vi "HFRR ADV v024 new software.vi"() -> ()   [LabVIEW 2025] (continued)
                n264 = local write "measured_stroke"(0.0 ("measured_stroke")) -> ()
                n265 = local write "Main Dashboard Buttons"(T1."Imaging" ("Main Dashboard Buttons")) -> ()
                n266 = property on="RUN" class="Bool (strict)"("Visible"=TRUE) -> ()  [unwired: 2 in, 2 out]
                n267 = local write "Due Write"("VC;0") -> ()
                n268 = local write "TEST FILE NAM,E SAVED"(FALSE ("TEST FILE NAM,E SAVED")) -> ()
                n269 = local write "Fuel Discription :"(w365) -> ()
                n270 = local write "Batch Ref Num :"(w365) -> ()
                n271 = local write "Remarks :"(w365) -> ()
                n272 = local write "FILE"(w365) -> ()
                n273 = property on="FRICVALZ 2" class="Bool (strict)"("DisabledEnum"=w364) -> ()  [unwired: 2 in, 2 out]
                n274 = property on="FRICVALZ 4" class="Bool (strict)"("DisabledEnum"=w364) -> ()  [unwired: 2 in, 2 out]
                n275 = property on="FRICVALZ 3" class="Bool (strict)"("DisabledEnum"=w364) -> ()  [unwired: 2 in, 2 out]
              }
            }
          }
          frame True {
            n276 = flat-sequence {
              frame #0 {
                n277 = local write "Due Write"("VC;1") -> ()
              }
              frame #1 {
                n278 = Wait (ms)(milliseconds to wait=u32 2000) -> ()  [unwired: 1 out]
              }
              frame #2 {
                n279 = local write "Due Write"("VC;1") -> ()
              }
              frame #3 {
                n280 = Wait (ms)(milliseconds to wait=u32 2000) -> ()  [unwired: 1 out]
              }
              frame #4 {
                w372 = T19."Disabled" ("Disabled")
                n281 = property on="RUN" class="Bool (strict)"("Visible"=FALSE) -> ()  [unwired: 2 in, 2 out]
                n282 = property on="FRICVALZ 2" class="Bool (strict)"("DisabledEnum"=w372) -> ()  [unwired: 2 in, 2 out]
                n283 = property on="FRICVALZ 4" class="Bool (strict)"("DisabledEnum"=w372) -> ()  [unwired: 2 in, 2 out]
                n284 = property on="FRICVALZ 3" class="Bool (strict)"("DisabledEnum"=w372) -> ()  [unwired: 2 in, 2 out]
                "START TEMP" <- TRUE
              }
            }
          }
        }
      }
      event "FILE", "USERNAME", "USER ID": Mouse Enter {
        n285 = event-data() -> ()  [unwired: 1 in, 4 out]
        n286 = dll-call lib="kernel32.dll" fn="Wow64DisableWow64FsRedirection"("OldValue"=0) -> (error out=w379:errorcluster, "OldValue"=w377:i32)  [unwired: 4 in, 1 out]
        n287 = call <vilib>:"System Exec.vi"("run minimized? (F)"=TRUE, "error in (no error)"=w379, "command line"="C:\\Program Files\\Common Files\\Microsoft Shared\\Ink\\TabTip.exe") -> ("error out"=w378:errorcluster)  [unwired: 5 in, 3 out]
        n288 = dll-call lib="kernel32.dll" fn="Wow64EnableWow64FsRedirection"(error in=w378, "OldValue"=w377) -> ()  [unwired: 4 in, 2 out]
      }
      event "EDIT": Value Change {
        n289 = event-data() -> ()  [unwired: 1 in, 6 out]
        n290 = local read "EDIT"() -> (w380:bool)
        n291 = case shown="False" w380 {
          frame False {
            n292 = control-ref of="This VI"() -> (w397:refnum<vi>)
            n293 = property class="VI"(reference=w397) -> (reference out=w388:refnum<vi>, error out=w392:errorcluster, "Panel"=w396:refnum<vi>)  [unwired: 1 in]
            n294 = property class="Pnl"(reference=w396, error in=w392) -> (reference out=w390:refnum<vi>, error out=w393:errorcluster, "Panes[]"=w395:refnum<vi>[])
            n295 = for {
              tunnel: w395 -> [w403] mode=indexing
              tunnel: T21."Always Off" ("Horizontal Scrollbar Visibility") -> [w402]
              tunnel: w393 -> [w399]
              tunnel: [w398] -> w391
              n296 = property class="Pane"(reference=w403, error in=w399, "HorizScrollbarVisibility"=w402) -> (reference out=w400:refnum<vi>, error out=w401:errorcluster)
              n297 = Close Reference(reference=w400, error in (no error)=w401) -> (error out=w398:errorcluster)
            }
            n298 = Close Reference(reference=w390, error in (no error)=w391) -> (error out=w389:errorcluster)
            n299 = Close Reference(reference=w388, error in (no error)=w389) -> (error out=w383:errorcluster)
            "error out 7" <- w383
            n300 = call <vilib>:"Clear Errors.vi"("error in (no error)"=w383) -> ("error out"=w382:errorcluster)  [unwired: 5 in, 1 out]
            n301 = local write "Service Password enable"(FALSE ("Service Password enable")) -> ()
            n302 = call <userlib>:"Fit VI window to Largest Dec.vi"("error in (no error)"=w382, "border spacing (2 px)"=1) -> ("error out"=w387:errorcluster, "dup VI Ref"=w385:refnum<vi>)  [unwired: 4 in]
            n303 = invoke on="Invoke Node" class="VI" method="FP.Run-Time Position.Maximized"(reference=w385, error in=w387) -> (error out=w386:errorcluster)  [unwired: 2 in, 3 out]
            n304 = call <vilib>:"Clear Errors.vi"("error in (no error)"=w386) -> ()  [unwired: 5 in, 2 out]
          }
          frame True {
          }
        }
      }
      event "Heater Button": Value Change {
        n305 = event-data() -> ()  [unwired: 1 in, 6 out]
        n306 = local read "Heater Button"() -> (w404:bool)
        n307 = case shown="True" w404 {
          frame True {
            n308 = stacked-sequence {
              frame #0 {
                n309 = Wait (ms)(milliseconds to wait=u32 1500) -> ()  [unwired: 1 out]
              }
              frame #1 {
                n310 = local read "Set Temp"() -> (w406:dbl)
                n311 = Number To Fractional String(number=w406, precision (6)=i16 2) -> (F-format string=w409:string)  [unwired: 2 in]
                n312 = Concatenate Strings("ST;" ("Command"), w409) -> (w408:string)
                n313 = local write "Due Write"(w408) -> ()
              }
              frame #2 {
                n314 = Wait (ms)(milliseconds to wait=u32 1500) -> ()  [unwired: 1 out]
              }
              frame #3 {
                n315 = local write "Due Write"("HE;1" ("Command")) -> ()
              }
              frame #4 {
                n316 = Wait (ms)(milliseconds to wait=u32 1500) -> ()  [unwired: 1 out]
              }
              frame #5 {
                n317 = stacked-sequence {
                  frame #0 {
                    n318 = Wait (ms)(milliseconds to wait=u32 1500) -> ()  [unwired: 1 out]
                  }
                  frame #1 {
                    n319 = local read "Set Temp"() -> (w415:dbl)
                    n320 = Number To Fractional String(number=w415, precision (6)=i16 2) -> (F-format string=w418:string)  [unwired: 2 in]
                    n321 = Concatenate Strings("ST;" ("Command"), w418) -> (w417:string)
                    n322 = local write "Due Write"(w417) -> ()
                  }
                  frame #2 {
                    n323 = Wait (ms)(milliseconds to wait=u32 1500) -> ()  [unwired: 1 out]
                  }
                  frame #3 {
                    n324 = local write "Due Write"("HE;1" ("Command")) -> ()
                  }
                  frame #4 {
                    n325 = Wait (ms)(milliseconds to wait=u32 1500) -> ()  [unwired: 1 out]
                  }
                }
              }
            }
          }
          frame False {
            n326 = stacked-sequence {
              frame #0 {
                n327 = Wait (ms)(milliseconds to wait=u32 1500) -> ()  [unwired: 1 out]
              }
              frame #1 {
                n328 = Concatenate Strings("ST;" ("Command"), "0" ("string")) -> (w425:string)
                n329 = local write "Due Write"(w425) -> ()
              }
              frame #2 {
                n330 = Wait (ms)(milliseconds to wait=u32 1500) -> ()  [unwired: 1 out]
              }
              frame #3 {
                n331 = local write "Due Write"("HE;0" ("Command")) -> ()
              }
              frame #4 {
                n332 = Wait (ms)(milliseconds to wait=u32 1500) -> ()  [unwired: 1 out]
              }
            }
          }
        }
      }
      event "Headen Service Button": Value Change {
        n333 = event-data() -> ()  [unwired: 1 in, 6 out]
        n334 = local read "Headen Service Button"() -> (w430:bool)
        n335 = case shown="True" w430 {
          frame False {
            n336 = property on="Password 3" class="Clust (strict)"("Visible"=FALSE) -> ()  [unwired: 2 in, 2 out]
            n337 = property on="Service Password Log" class="Str"("Visible"=FALSE) -> ()  [unwired: 2 in, 2 out]
          }
          frame True {
            n338 = property on="Password 3" class="Clust (strict)"("Visible"=TRUE) -> ()  [unwired: 2 in, 2 out]
            n339 = property on="Service Password Log" class="Str"("Visible"=TRUE) -> ()  [unwired: 2 in, 2 out]
          }
        }
      }
      event "Password 3.Service Password": Value Change {
        n340 = event-data() -> ()  [unwired: 1 in, 6 out]
        n341 = Unbundle By Name("Password 3") -> ("Service Password"=w437:string)
        n342 = call <vilib>:"Trim Whitespace.vi"("string"=w437) -> ("trimmed string"=w435:string)  [unwired: 1 in]
        n343 = Equal?(x=w435, y="Service@123") -> (x = y?=w436:bool)
        n344 = case shown="False" w436 {
          selector: w436 -> [w441 w443]
          frame False {
            n345 = local write "Service Password enable"(w441) -> ()
            n346 = property on="Service Password Log" class="Str"("Visible"=TRUE) -> ()  [unwired: 2 in, 2 out]
            n347 = property on="Tab Control 5" class="TabCtl (strict)"("Tabs Visible?"=TRUE ("Page Labels Display Visible?")) -> ()  [unwired: 2 in, 2 out]
          }
          frame True {
            n348 = property on="Service Password Log" class="Str"("Visible"=FALSE) -> ()  [unwired: 2 in, 2 out]
            "Service Password enable" <- w443
          }
        }
      }
      event "Sign In": Value Change {
        w445 = FALSE ("Visible")
        n349 = event-data() -> ()  [unwired: 1 in, 6 out]
        n350 = property on="About" class="Clust (strict)"("Visible"=w445) -> ()  [unwired: 2 in, 2 out]
        n351 = property on="Password 3" class="Clust (strict)"("Visible"=w445) -> ()  [unwired: 2 in, 2 out]
        n352 = property on="Service Password Log" class="Str"("Visible"=FALSE) -> ()  [unwired: 2 in, 2 out]
      }
      event "Info": Value Change {
        n353 = event-data() -> ()  [unwired: 1 in, 6 out]
        n354 = local read "Info"() -> (w447:bool)
        n355 = case shown="False" w447 {
          frame False {
            n356 = property on="About" class="Clust (strict)"("Visible"=FALSE) -> ()  [unwired: 2 in, 2 out]
          }
          frame True {
            n357 = property on="About" class="Clust (strict)"("Visible"=TRUE) -> ()  [unwired: 2 in, 2 out]
          }
        }
      }
      event "Calibration": Value Change {
        n358 = event-data() -> ()  [unwired: 1 in, 6 out]
        n359 = local read "Calibration"() -> (w451:bool)
        n360 = case shown="False" w451 {
          frame False {
            n361 = property on="Calibration 2" class="TabCtl (strict)"("Visible"=FALSE) -> ()  [unwired: 2 in, 2 out]
            n362 = local write "Cal Password"("" ("Cal Password")) -> ()
          }
          frame True {
            n363 = property on="Calibration 2" class="TabCtl (strict)"("Visible"=TRUE) -> ()  [unwired: 2 in, 2 out]
            n364 = local write "Cal Password"("" ("Cal Password")) -> ()
          }
        }
        n365 = property on="Wrong Password" class="Str"("Visible"=FALSE) -> ()  [unwired: 2 in, 2 out]
      }
      event "Cal Password": Value Change {
        n366 = event-data() -> ()  [unwired: 1 in, 6 out]
        n367 = local read "Cal Password"() -> (w459:string)
        n368 = call <vilib>:"Trim Whitespace.vi"("string"=w459) -> ("trimmed string"=w458:string)  [unwired: 1 in]
        n369 = Equal?(x=w458, y="Cal@321") -> (x = y?=w456:bool)
        n370 = case shown="True" w456 {
          frame False {
            n371 = property on="Wrong Password" class="Str"("Visible"=TRUE) -> ()  [unwired: 2 in, 2 out]
          }
          frame True {
            n372 = property on="Wrong Password" class="Str"("Visible"=FALSE) -> ()  [unwired: 2 in, 2 out]
            n373 = local write "Main Tab"(T2."About" ("Main Tab")) -> ()
            n374 = local write "Cal Password"("" ("Cal Password")) -> ()
            n375 = local write "Main Dashboard Buttons"(T1."About" ("Main Dashboard Buttons")) -> ()
            n376 = local write "Tab Control 5"(T12."Temperature Calibration" ("Tab Control 5")) -> ()
            n377 = property on="Calibration 2" class="TabCtl (strict)"("Visible"=FALSE) -> ()  [unwired: 2 in, 2 out]
            n378 = property on="Tab Control 5" class="TabCtl (strict)"("Tabs Visible?"=FALSE ("Page Labels Display Visible?")) -> ()  [unwired: 2 in, 2 out]
            n379 = local write "Calibration"(FALSE ("Calibration")) -> ()
          }
        }
      }
      event "Calibration Selection": Value Change {
        n380 = event-data() -> ()  [unwired: 1 in, 6 out]
        n381 = local read "Calibration Selection"() -> (w470:T8)
        n382 = case shown="\"Stroke Calibration\"" w470 {
          tunnel: [T7."Stroke" ("Main Calibration Tab") T7."Friction" ("Main Calibration Tab") T7."Main" ("Main Calibration Tab") T7."Temperature" ("Main Calibration Tab")] -> w469
          frame "Stroke Calibration" {
          }
          frame "Friction Force Calibration" {
          }
          frame Default {
          }
          frame "Temperature Calibration" {
          }
        }
        n383 = local write "Main Calibration Tab"(w469) -> ()
      }
      event "Back Stroke": Value Change {
        n384 = event-data() -> ()  [unwired: 1 in, 6 out]
        n385 = local write "Main Stroke Tab"(T9."Step 1" ("Main Stroke Tab")) -> ()
        n386 = local write "Main Calibration Tab"(T7."Main" ("Main Calibration Tab")) -> ()
        n387 = local write "Back Stroke"(FALSE ("Back Stroke")) -> ()
      }
      event "Step 2 Back": Value Change {
        n388 = event-data() -> ()  [unwired: 1 in, 6 out]
        n389 = local write "Main Stroke Tab"(T9."Step 1" ("Main Stroke Tab")) -> ()
        n390 = local write "Step 2 Back"(FALSE ("Back Stroke")) -> ()
      }
      event "Step 3 Back": Value Change {
        n391 = event-data() -> ()  [unwired: 1 in, 6 out]
        n392 = local write "Main Stroke Tab"(T9."Step 2" ("Main Stroke Tab")) -> ()
        n393 = local write "Step 3 Back"(FALSE ("Back Stroke")) -> ()
      }
      event "Step 4 Back": Value Change {
        n394 = event-data() -> ()  [unwired: 1 in, 6 out]
        n395 = local write "Main Stroke Tab"(T9."Step 3" ("Main Stroke Tab")) -> ()
        n396 = local write "Step 4 Back"(FALSE ("Back Stroke")) -> ()
      }
      event "Step 5 Back": Value Change {
        n397 = event-data() -> ()  [unwired: 1 in, 6 out]
        n398 = local write "Main Stroke Tab"(T9."Step 4" ("Main Stroke Tab")) -> ()
        n399 = local write "Step 5 Back"(FALSE ("Back Stroke")) -> ()
      }
      event "Step 6 Back": Value Change {
        n400 = event-data() -> ()  [unwired: 1 in, 6 out]
        n401 = local write "Main Stroke Tab"(T9."Step 5" ("Main Stroke Tab")) -> ()
        n402 = local write "Step 6 Back"(FALSE ("Back Stroke")) -> ()
      }
      event "Back Stroke step 7": Value Change {
        n403 = event-data() -> ()  [unwired: 1 in, 6 out]
        n404 = local write "Main Stroke Tab"(T9."Step 6" ("Main Stroke Tab")) -> ()
        n405 = local write "Back Stroke step 7"(FALSE ("Back Stroke")) -> ()
      }
      event "Back Stroke step 8": Value Change {
        n406 = event-data() -> ()  [unwired: 1 in, 6 out]
        n407 = local write "Main Stroke Tab"(T9."Step 7" ("Main Stroke Tab")) -> ()
        n408 = local write "Back Stroke step 8"(FALSE ("Back Stroke")) -> ()
      }
      event "Back Stroke 8": Value Change {
        n409 = event-data() -> ()  [unwired: 1 in, 6 out]
        n410 = local write "MOVE CARRIAGE TO"(0.2 ("MOVE CARRIAGE TO")) -> ()
        n411 = local write "Main Stroke Tab"(T9."Step 1" ("Main Stroke Tab")) -> ()
        n412 = local write "Back Stroke 8"(FALSE ("Back Stroke 8")) -> ()
      }
      event "Continue Stroke": Value Change {
        n413 = event-data() -> ()  [unwired: 1 in, 6 out]
        n414 = local write "Main Stroke Tab"(T9."Step 2" ("Main Stroke Tab")) -> ()
        n415 = local write "Continue Stroke"(FALSE ("Continue Stroke")) -> ()
      }
      event "Continue Stroke step 2": Value Change {
        n416 = event-data() -> ()  [unwired: 1 in, 6 out]
        n417 = local write "Main Stroke Tab"(T9."Step 3" ("Main Stroke Tab")) -> ()
        n418 = local write "Continue Stroke step 2"(FALSE ("Continue Stroke")) -> ()
      }
      event "Continue Stroke step 3": Value Change {
        n419 = event-data() -> ()  [unwired: 1 in, 6 out]
        n420 = local write "Main Stroke Tab"(T9."Step 4" ("Main Stroke Tab")) -> ()
        n421 = local write "Continue Stroke step 3"(FALSE ("Continue Stroke")) -> ()
      }
      event "Continue Stroke step 4": Value Change {
        n422 = event-data() -> ()  [unwired: 1 in, 6 out]
        n423 = local write "Main Stroke Tab"(T9."Step 5" ("Main Stroke Tab")) -> ()
        n424 = local write "Continue Stroke step 4"(FALSE ("Continue Stroke")) -> ()
      }
      event "Continue Stroke step 5": Value Change {
        n425 = event-data() -> ()  [unwired: 1 in, 6 out]
        n426 = local write "Main Stroke Tab"(T9."Step 6" ("Main Stroke Tab")) -> ()
        n427 = local write "Continue Stroke step 5"(FALSE ("Continue Stroke")) -> ()
      }
      event "Continue Stroke step 6": Value Change {
        n428 = event-data() -> ()  [unwired: 1 in, 6 out]
        n429 = local write "Main Stroke Tab"(T9."Step 7" ("Main Stroke Tab")) -> ()
        n430 = local write "Continue Stroke step 6"(FALSE ("Continue Stroke")) -> ()
      }
      event "Continue Stroke step 7": Value Change {
        w509 = FALSE ("0.2mm")
        n431 = event-data() -> ()  [unwired: 1 in, 6 out]
        n432 = local write "0.4 mm"(w509) -> ()
        n433 = local write "0.6 mm"(w509) -> ()
        n434 = local write "1.0 mm"(w509) -> ()
        n435 = local write "1.2 mm"(w509) -> ()
        n436 = local write "0.2 2"(w509) -> ()
        n437 = local write "0.4 2"(w509) -> ()
        n438 = local write "0.6 2"(w509) -> ()
        n439 = local write "0.8 2"(w509) -> ()
        n440 = local write "1.0 2"(w509) -> ()
        n441 = local write "1.2"(w509) -> ()
        n442 = local write "0.2mm"(w509) -> ()
        n443 = local write "0.8mm"(w509) -> ()
        n444 = local write "Main Stroke Tab"(T9."Step 8" ("Main Stroke Tab")) -> ()
        n445 = local write "Continue Stroke step 7"(FALSE ("Continue Stroke")) -> ()
        n446 = local write "Stroke Test Complete"(T10."Test Progress" ("Stroke Test Complete")) -> ()
        "Position Measurment Temp" <- 0.0 ("Position Measurment Temp")
        "Calibration Tare" <- TRUE ("Calibration Tare")
        "MOVE CARRIAGE TO" <- 0.2 ("MOVE CARRIAGE TO")
      }
      event "Continue Stroke step 8": Value Change {
        n447 = event-data() -> ()  [unwired: 1 in, 6 out]
        n448 = local read "LVDT STROKE  Calibration"() -> (w514:dbl)
        n449 = local read "Position Measurment Temp"() -> (w515:dbl)
        n450 = case shown="7" w515 {
          selector: w515 -> [w520 w525 w530 w535 w540 w544 w547 w548]
          tunnel: w514 -> [w516 w521 w526 w531 w536 w541 _ _]
          frame 0, Default {
            w518 = TRUE ("0.2mm")
            n451 = Increment(x=w520) -> (x+1=w519:i32)
            n452 = local write "Position Measurment Temp"(w519) -> ()
            n453 = local write "0.2mm"(w518) -> ()
            n454 = local write "0.2 2"(w518) -> ()
            n455 = local write "MOVE CARRIAGE TO"(0.4 ("MOVE CARRIAGE TO")) -> ()
            "Calibration 0.2" <- w516
          }
          frame 1 {
            w523 = TRUE ("0.4 mm")
            n456 = Increment(x=w525) -> (x+1=w524:i32)
            n457 = local write "Calibration 0.4"(w521) -> ()
            n458 = local write "Position Measurment Temp"(w524) -> ()
            n459 = local write "0.4 mm"(w523) -> ()
            n460 = local write "MOVE CARRIAGE TO"(0.6 ("MOVE CARRIAGE TO")) -> ()
            n461 = local write "0.4 2"(w523) -> ()
          }
          frame 2 {
            w528 = TRUE ("0.6 mm")
            n462 = Increment(x=w530) -> (x+1=w529:i32)
            n463 = local write "Calibration 0.6"(w526) -> ()
            n464 = local write "Position Measurment Temp"(w529) -> ()
            n465 = local write "0.6 2"(w528) -> ()
            n466 = local write "0.6 mm"(w528) -> ()
            n467 = local write "MOVE CARRIAGE TO"(0.8 ("MOVE CARRIAGE TO")) -> ()
          }
          frame 3 {
            w532 = TRUE ("0.6 mm")
            n468 = Increment(x=w535) -> (x+1=w534:i32)
            n469 = local write "Position Measurment Temp"(w534) -> ()
            n470 = local write "MOVE CARRIAGE TO"(1.0 ("MOVE CARRIAGE TO")) -> ()
            n471 = local write "0.8mm"(w532) -> ()
            n472 = local write "0.8 2"(w532) -> ()
            "Calibration 0.8" <- w531
          }
          frame 4 {
            w537 = TRUE ("0.6 mm")
            n473 = Increment(x=w540) -> (x+1=w539:i32)
            n474 = local write "Position Measurment Temp"(w539) -> ()
            n475 = local write "MOVE CARRIAGE TO"(1.2 ("MOVE CARRIAGE TO")) -> ()
            n476 = local write "1.0 mm"(w537) -> ()
            n477 = local write "1.0 2"(w537) -> ()
            "Calibration 1.0" <- w536
          }
          frame 5 {
            w542 = TRUE ("0.6 mm")
            n478 = Increment(x=w544) -> (x+1=w543:i32)
            n479 = local write "Position Measurment Temp"(w543) -> ()
            n480 = local write "1.2 mm"(w542) -> ()
            n481 = local write "1.2"(w542) -> ()
            "Calibration 1.2" <- w541
          }
          frame 6 {
            n482 = Increment(x=w547) -> (x+1=w546:i32)
            n483 = local write "Position Measurment Temp"(w546) -> ()
            n484 = local write "Stroke Test Complete"(T10."Stroke Points Completed" ("Stroke Test Complete")) -> ()
          }
          frame 7 {
            n485 = stacked-sequence {
              tunnel: w548 -> [w549 _ _]
              frame #0 {
                n486 = Increment(x=w549) -> (x+1=w550:i32)
                n487 = local write "Main Stroke Tab"(T9."Step 9" ("Main Stroke Tab")) -> ()
                n488 = local write "Position Measurment Temp"(w550) -> ()
                n489 = Insert Into Array(array=dbl[] [], new element #1=0.2 ("new element/subarray"), new element #2=0.4 ("new element/subarray"), new element #3=0.6 ("new element/subarray"), new element #4=0.8 ("new element/subarray"), new element #5=1.0 ("new element/subarray"), new element #6=1.2 ("new element/subarray")) -> (→"1D stroke":dbl[])  [unwired: 1 in]
                n490 = local read "Calibration 0.2"() -> (w557:dbl)
                n491 = local read "Calibration 0.4"() -> (w556:dbl)
                n492 = local read "Calibration 0.6"() -> (w555:dbl)
                n493 = local read "Calibration 0.8"() -> (w554:dbl)
                n494 = local read "Calibration 1.0"() -> (w553:dbl)
                n495 = local read "Calibration 1.2"() -> (w552:dbl)
                n496 = Insert Into Array(array=dbl[] [], new element #1=w557, new element #2=w556, new element #3=w555, new element #4=w554, new element #5=w553, new element #6=w552) -> (→"Calibrated Voltage Value":dbl[])  [unwired: 1 in]
              }
              frame #1 {
                n497 = local read "calibration values"() -> (w580:dbl[])
                n498 = local read "Calibrated Voltage Value"() -> (w582:dbl[])
                n499 = Index Array(array=w580, index #1=1 ("index"), index #2=3 ("index"), index #3=5 ("index"), index #4=7 ("index"), index #5=9 ("index"), index #6=11 ("index")) -> (element #1=w573:dbl, element #2=w572:dbl, element #3=w571:dbl, element #4=w570:dbl, element #5=w569:dbl, element #6=w568:dbl)
                n500 = local read "1D stroke"() -> (w583:dbl[])
                n501 = for {
                  tunnel: [w592] -> w581 mode=indexing
                  tunnel: w583 -> [w591] mode=indexing
                  tunnel: w582 -> [w590] mode=indexing
                  tunnel: w573 -> [w589]
                  tunnel: w572 -> [w588]
                  tunnel: w571 -> [w587]
                  tunnel: w570 -> [w586]
                  tunnel: w569 -> [w585]
                  tunnel: w568 -> [w584]
                  n502 = formula code="if (stroke == 0.2)\n{\n    if ((voltage >= REF_02 * 0.985) && (voltage <= REF_02 * 1.015))\n        status = 1;\n    else\n        status = 0;\n}\nelse if (stroke == 0.4)\n{\n    if ((voltage >= REF_04 * 0.985) && (voltage <= REF_04 * 1.015))\n        status = 1;\n    else\n        status = 0;\n}\nelse if (stroke == 0.6)\n{\n    if ((voltage >= REF_06 * 0.985) && (voltage <= REF_06 * 1.015))\n        status = 1;\n    else\n        status = 0;\n}\nelse if (stroke == 0.8)\n{\n    if ((voltage >= REF_08 * 0.985) && (voltage <= REF_08 * 1.015))\n        status = 1;\n    else\n        status = 0;\n}\nelse if (stroke == 1.0)\n{\n    if ((voltage >= REF_10 * 0.985) && (voltage <= REF_10 * 1.015))\n        status = 1;\n    else\n        status = 0;\n}\nelse if (stroke == 1.2)\n{\n    if ((voltage >= REF_12 * 0.985) && (voltage <= REF_12 * 1.015))\n        status = 1;\n    else\n        status = 0;\n}\nelse\n{\n    status = 0;\n}"("stroke"=w591, "voltage"=w590, "REF_02"=w589, "REF_04"=w588, "REF_06"=w587, "REF_08"=w586, "REF_10"=w585, "REF_12"=w584) -> ("status"=w592:dbl)
                }
                "Status" <- w581
              }
              frame #2 {
                w599 = 1.0
                n503 = local read "Status"() -> (w606:dbl[])
                n504 = Index Array(array=w606) -> (element #1=w605:dbl, element #2=w604:dbl, element #3=w603:dbl, element #4=w602:dbl, element #5=w601:dbl, element #6=w600:dbl)  [unwired: 6 in]
                n505 = Equal?(x=w604, y=w599) -> (x = y?=w597:bool)
                n506 = Equal?(x=w603, y=w599) -> (x = y?=w596:bool)
                n507 = Equal?(x=w602, y=w599) -> (x = y?=w595:bool)
                n508 = Equal?(x=w601, y=w599) -> (x = y?=w594:bool)
                n509 = Equal?(x=w600, y=w599) -> (x = y?=w593:bool)
                n510 = Equal?(x=w605, y=w599) -> (x = y?=w598:bool)
                n511 = case shown="True" w598 {
                  selector: w598 -> [w617 w618]
                  frame True {
                    n512 = local write "Point 1 - 0.2 mm"(w617) -> ()
                    n513 = property on="Point 1 - 0.2 mm" class="Bool"("Caption.Visible"=w617) -> ()  [unwired: 2 in, 2 out]
                  }
                  frame False {
                    n514 = local write "Point 1 - 0.2 mm"(w618) -> ()
                    n515 = property on="Point 1 - 0.2 mm" class="Bool"("Caption.Visible"=w618) -> ()  [unwired: 2 in, 2 out]
                  }
                }
                n516 = case shown="True" w597 {
                  selector: w597 -> [w615 w616]
                  frame True {
                    n517 = local write "Point 2 - 0.4 mm"(w615) -> ()
                    n518 = property on="Point 2 - 0.4 mm" class="Bool"("Caption.Visible"=w615) -> ()  [unwired: 2 in, 2 out]
                  }
                  frame False {
                    n519 = local write "Point 2 - 0.4 mm"(w616) -> ()
                    n520 = property on="Point 2 - 0.4 mm" class="Bool"("Caption.Visible"=w616) -> ()  [unwired: 2 in, 2 out]
                  }
                }
                n521 = case shown="True" w594 {
                  selector: w594 -> [w609 w610]
                  frame True {
                    n522 = local write "Point 5 - 1.0 mm"(w609) -> ()
                    n523 = property on="Point 5 - 1.0 mm" class="Bool"("Caption.Visible"=w609) -> ()  [unwired: 2 in, 2 out]
                  }
                  frame False {
                    n524 = local write "Point 5 - 1.0 mm"(w610) -> ()
                    n525 = property on="Point 5 - 1.0 mm" class="Bool"("Caption.Visible"=w610) -> ()  [unwired: 2 in, 2 out]
                  }
                }
                n526 = case shown="True" w596 {
                  selector: w596 -> [w613 w614]
                  frame True {
                    n527 = local write "Point 3 - 0.6 mm"(w613) -> ()
                    n528 = property on="Point 3 - 0.6 mm" class="Bool"("Caption.Visible"=w613) -> ()  [unwired: 2 in, 2 out]
                  }
                  frame False {
                    n529 = local write "Point 3 - 0.6 mm"(w614) -> ()
                    n530 = property on="Point 3 - 0.6 mm" class="Bool"("Caption.Visible"=w614) -> ()  [unwired: 2 in, 2 out]
                  }
                }
                n531 = case shown="True" w595 {
                  selector: w595 -> [w611 w612]
                  frame True {
                    n532 = local write "Point 4 - 0.8 mm"(w611) -> ()
                    n533 = property on="Point 4 - 0.8 mm" class="Bool"("Caption.Visible"=w611) -> ()  [unwired: 2 in, 2 out]
                  }
                  frame False {
                    n534 = local write "Point 4 - 0.8 mm"(w612) -> ()
                    n535 = property on="Point 4 - 0.8 mm" class="Bool"("Caption.Visible"=w612) -> ()  [unwired: 2 in, 2 out]
                  }
                }
                n536 = case shown="True" w593 {
                  selector: w593 -> [w607 w608]
                  frame True {
                    n537 = local write "Point 6 - 1.2 mm"(w607) -> ()
                    n538 = property on="Point 6 - 1.2 mm" class="Bool"("Caption.Visible"=w607) -> ()  [unwired: 2 in, 2 out]
                  }
                  frame False {
                    n539 = local write "Point 6 - 1.2 mm"(w608) -> ()
                    n540 = property on="Point 6 - 1.2 mm" class="Bool"("Caption.Visible"=w608) -> ()  [unwired: 2 in, 2 out]
                  }
                }
              }
            }
          }
        }
      }
      event "TEMPERATURE STEP Back 1", "TEMPERATURE STEP Back air Temp": Value Change {
        n541 = event-data() -> ()  [unwired: 1 in, 6 out]
        n542 = stacked-sequence {
          frame #0 {
            n543 = local write "Main Calibration Tab"(T7."Main" ("Main Calibration Tab")) -> ()
          }
          frame #1 {
            n544 = Wait (ms)(milliseconds to wait=u32 1000) -> ()  [unwired: 1 out]
          }
          frame #2 {
            n545 = local write "Due Write"("CAL;END" ("Command")) -> ()
          }
          frame #3 {
            n546 = Wait (ms)(milliseconds to wait=u32 2000) -> ()  [unwired: 1 out]
          }
          frame #4 {
            n547 = local write "Due Write"("CAL;END" ("Command")) -> ()
          }
        }
      }
      event "Temperature Continue Step 1": Value Change {
        n548 = event-data() -> ()  [unwired: 1 in, 6 out]
        n549 = stacked-sequence {
          frame #0 {
            n550 = Wait (ms)(milliseconds to wait=u32 1500) -> ()  [unwired: 1 out]
          }
          frame #1 {
            n551 = local write "Due Write"("CAL;START" ("Command")) -> ()
          }
          frame #2 {
            n552 = Wait (ms)(milliseconds to wait=u32 1500) -> ()  [unwired: 1 out]
          }
          frame #3 {
            n553 = local write "Due Write"("CAL;START" ("Command")) -> ()
          }
          frame #4 {
            n554 = Wait (ms)(milliseconds to wait=u32 2000) -> ()  [unwired: 1 out]
          }
          frame #5 {
          }
          frame #6 {
            n555 = Wait (ms)(milliseconds to wait=u32 2000) -> ()  [unwired: 1 out]
          }
          frame #7 {
            # "CAL;A1;<true_T>"
            n556 = local write "Due Write"("CAL;A1;0" ("Command")) -> ()
          }
          frame #8 {
            n557 = local write "Tab Control 4"(T11."Step 2" ("Tab Control 4")) -> ()
          }
        }
      }
      event "Temperature Continue Step air Step 1": Value Change {
        n558 = event-data() -> ()  [unwired: 1 in, 6 out]
        n559 = stacked-sequence {
          frame #0 {
            n560 = Wait (ms)(milliseconds to wait=u32 1500) -> ()  [unwired: 1 out]
          }
          frame #1 {
            n561 = local write "Due Write"("CAL;START" ("Command")) -> ()
          }
          frame #2 {
            n562 = local write "Tab Control 4"(T11."Air Step 2" ("Tab Control 4")) -> ()
            n563 = Wait (ms)(milliseconds to wait=u32 1500) -> ()  [unwired: 1 out]
          }
          frame #3 {
            n564 = local write "Due Write"("CAL;START" ("Command")) -> ()
          }
          frame #4 {
            n565 = Wait (ms)(milliseconds to wait=u32 2000) -> ()  [unwired: 1 out]
          }
          frame #5 {
            # "CAL;A1;<true_T>"
            n566 = local write "Due Write"("CAL;A2;0" ("Command")) -> ()
          }
          frame #6 {
            n567 = Wait (ms)(milliseconds to wait=u32 2000) -> ()  [unwired: 1 out]
          }
          frame #7 {
            # "CAL;A1;<true_T>"
            n568 = local write "Due Write"("CAL;A1;0" ("Command")) -> ()
          }
        }
      }
      event "Temperature Selection": Value Change {
        n569 = event-data() -> ()  [unwired: 1 in, 6 out]
        n570 = local read "Temperature Selection"() -> (w641:enum32{"Air Temperature", "Sample Temperature"})
        n571 = case shown="\"Sample Temperature\"" w641 {
          frame "Air Temperature", Default {
            n572 = local write "Tab Control 4"(T11."Air Step 1" ("Tab Control 4")) -> ()
          }
          frame "Sample Temperature" {
            n573 = local write "Tab Control 4"(T11."Step 1" ("Tab Control 4")) -> ()
          }
        }
      }
      event "Temperature Continue Step 2": Value Change {
        n574 = event-data() -> ()  [unwired: 1 in, 6 out]
        n575 = stacked-sequence {
          frame #0 {
            n576 = stacked-sequence {
              frame #0 {
                n577 = Wait (ms)(milliseconds to wait=u32 1500) -> ()  [unwired: 1 out]
              }
              frame #1 {
                # "CAL;A1;<true_T>"
                n578 = local write "Due Write"("CAL;A1;0" ("Command")) -> ()
              }
              frame #2 {
                n579 = Wait (ms)(milliseconds to wait=u32 1500) -> ()  [unwired: 1 out]
              }
              frame #3 {
                # "CAL;A1;<true_T>"
                n580 = local write "Due Write"("CAL;A1;0" ("Command")) -> ()
              }
              frame #4 {
              }
            }
          }
          frame #1 {
            n581 = local write "Tab Control 4"(T11."Step 3" ("Tab Control 4")) -> ()
          }
        }
      }
      event "Temperature Continue Step 3": Value Change {
        n582 = event-data() -> ()  [unwired: 1 in, 6 out]
        n583 = stacked-sequence {
          frame #0 {
            n584 = stacked-sequence {
              frame #0 {
                n585 = Wait (ms)(milliseconds to wait=u32 1500) -> ()  [unwired: 1 out]
              }
              frame #1 {
              }
              frame #2 {
              }
              frame #3 {
                # "CAL;A1;<true_T>"
                n586 = local write "Due Write"("CAL;A1;60" ("Command")) -> ()
              }
              frame #4 {
                n587 = Wait (ms)(milliseconds to wait=u32 2000) -> ()  [unwired: 1 out]
              }
              frame #5 {
                # "CAL;A1;<true_T>"
                n588 = local write "Due Write"("CAL;A1;60" ("Command")) -> ()
              }
            }
          }
          frame #1 {
            n589 = Wait (ms)(milliseconds to wait=u32 1000) -> ()  [unwired: 1 out]
          }
          frame #2 {
            n590 = local write "Due Write"("CAL;SAVE" ("Command")) -> ()
          }
          frame #3 {
            n591 = Wait (ms)(milliseconds to wait=u32 1000) -> ()  [unwired: 1 out]
          }
          frame #4 {
            n592 = local write "Due Write"("CAL;SAVE" ("Command")) -> ()
          }
          frame #5 {
            n593 = Wait (ms)(milliseconds to wait=u32 1000) -> ()  [unwired: 1 out]
          }
          frame #6 {
            # "CAL;END"
            n594 = local write "Due Write"("CAL;END" ("Command")) -> ()
          }
          frame #7 {
            n595 = Wait (ms)(milliseconds to wait=u32 1000) -> ()  [unwired: 1 out]
          }
          frame #8 {
            # "CAL;END"
            n596 = local write "Due Write"("CAL;END" ("Command")) -> ()
          }
          frame #9 {
            n597 = local write "Main Calibration Tab"(T7."Temperature" ("Main Calibration Tab")) -> ()
            n598 = local write "Tab Control 4"(T11."Main" ("Tab Control 4")) -> ()
          }
        }
      }
      event "Back Stroke step main temperature": Value Change {
        n599 = event-data() -> ()  [unwired: 1 in, 6 out]
        n600 = stacked-sequence {
          frame #0 {
            n601 = Wait (ms)(milliseconds to wait=u32 1000) -> ()  [unwired: 1 out]
          }
          frame #1 {
            # "CAL;END"
            n602 = local write "Due Write"("CAL;END" ("Command")) -> ()
          }
          frame #2 {
            n603 = Wait (ms)(milliseconds to wait=u32 1000) -> ()  [unwired: 1 out]
          }
          frame #3 {
            # "CAL;END"
            n604 = local write "Due Write"("CAL;END" ("Command")) -> ()
          }
          frame #4 {
            n605 = local write "Main Calibration Tab"(T7."Temperature" ("Main Calibration Tab")) -> ()
            n606 = local write "Tab Control 4"(T11."Main" ("Tab Control 4")) -> ()
          }
        }
      }
      event "Quit": Value Change {
        n607 = event-data() -> ()  [unwired: 1 in, 6 out]
      }
    }
    n608 = Wait (ms)(milliseconds to wait=u32 100) -> ()  [unwired: 1 out]
  }
  n609 = while {
    stop <- w674 stop-if-true
    n610 = local read "Ambient Temperature"() -> (w672:dbl)
    n611 = local read "Sample Temperature"() -> (w671:dbl)
    n612 = Wait (ms)(milliseconds to wait=u32 200) -> ()  [unwired: 1 out]
    n613 = local write "Temperature — Live (Set A: 0 °C)"(w672) -> ()
    n614 = local write "Temperature — Live (Set A: 60 °C)"(w672) -> ()
    n615 = local write "Sensor value"(w672) -> ()
    n616 = local write "Sensor value"(w672) -> ()
    n617 = local write "Sensor value"(w671) -> ()
    n618 = local write "Sensor value"(w671) -> ()
    n619 = local write "Temperature — Live (Set A: 60 °C)"(w671) -> ()
    n620 = local write "Temperature — Live (Set A: 60 °C)"(w671) -> ()
    n621 = case shown="True" "Save Button" {
      selector: "Save Button" -> [_ w676]
      frame False {
      }
      frame True {
        n622 = Not(x=w676) -> (.not. x?=w675:bool)
        n623 = local read "milliseconds to wait"() -> (w708:u32)
        n624 = local read "max_step_change"() -> (w713:dbl)
        n625 = local read "max_amplitude"() -> (w714:dbl)
        n626 = local read "min_amplitude"() -> (w715:dbl)
        n627 = local read "PIEZO_CAL_FACTOR"() -> (w719:dbl)
        n628 = local write "Save Button"(w675) -> ()
        n629 = local read "startup_cmd"() -> (w716:dbl)
        n630 = local read "NORMAL_FORCE"() -> (w720:dbl)
        n631 = local read "ADC_Resolution"() -> (w718:dbl)
        n632 = local read "calibration values"() -> (w723:dbl[])
        n633 = local read "kp"() -> (w710:dbl)
        n634 = local read "kd"() -> (w712:dbl)
        n635 = local read "dt"() -> (w709:dbl)
        n636 = local read "ki"() -> (w711:dbl)
        n637 = local read "STROKE FILTER"() -> (w721:i32)
        n638 = local read "Add up Stroke"() -> (w722:dbl)
        n639 = local read "VREF"() -> (w717:dbl)
        n640 = Insert Into Array(array=dbl[] [], new element #1=w708, new element #2=w709, new element #3=w710, new element #4=w711, new element #5=w712, new element #6=w713, new element #7=w714, new element #8=w715, new element #9=w716) -> (w724:dbl[])  [unwired: 1 in]
        n641 = Insert Into Array(array=dbl[] [], new element #1=w717, new element #2=w718, new element #3=w719, new element #4=w720) -> (w725:dbl[])  [unwired: 1 in]
        n642 = Array To Spreadsheet String(delimiter (Tab)=";", array=w723, 3:"" ("format string")) -> (spreadsheet string=w727:string)
        n643 = Insert Into Array(array=dbl[] [], new element #1=w721, new element #2=w722) -> (w726:dbl[])  [unwired: 1 in]
        n644 = call "Write Config.vi"("Stroke Calibration"=w727, "STROKE PARAMETERS"=w726, "ADC PARAMETERS"=w725, "PID  PARAMETERS"=w724) -> ("error out"=w706:errorcluster)  [unwired: 7 in]
        n645 = call "Stall Data Flow.vim"("value in"=w706, "milliseconds to wait"=u32 2000) -> ("value out"=w707:errorcluster)  [unwired: 1 out]
        n646 = call "Read Config.vi"("error in (no error)"=w707) -> ("STROKE PARAMETERS"=w704:dbl[], "ADC PARAMETERS"=w703:dbl[], "PID  PARAMETERS"=w702:dbl[], "Stroke Calibration"=w705:string)  [unwired: 6 in, 1 out]
        n647 = Index Array(array=w702) -> (element #1=w700:dbl, element #2=w699:dbl, element #3=w698:dbl, element #4=w697:dbl, element #5=w696:dbl, element #6=w695:dbl, element #7=w694:dbl, element #8=w693:dbl, element #9=w692:dbl)  [unwired: 9 in]
        n648 = Index Array(array=w703) -> (element #1=w691:dbl, element #2=w690:dbl, element #3=w689:dbl, element #4=w688:dbl)  [unwired: 4 in]
        n649 = Index Array(array=w704) -> (element #1=w687:dbl, element #2=w686:dbl)  [unwired: 2 in]
        n650 = Spreadsheet String To Array(delimiter (Tab)=";", format string="", spreadsheet string=w705, array type (2D Dbl)=dbl[] []) -> (array=w701:dbl[])
        n651 = local write "VREF"(w691) -> ()
        n652 = local write "ADC_Resolution"(w690) -> ()
        n653 = local write "PIEZO_CAL_FACTOR"(w689) -> ()
        n654 = local write "NORMAL_FORCE"(w688) -> ()
        n655 = local write "STROKE FILTER"(w687) -> ()
        n656 = local write "Add up Stroke"(w686) -> ()
        n657 = local write "calibration values"(w701) -> ()
        n658 = local write "milliseconds to wait"(w700) -> ()
        n659 = local write "dt"(w699) -> ()
        n660 = local write "kp"(w698) -> ()
        n661 = local write "ki"(w697) -> ()
        n662 = local write "kd"(w696) -> ()
        n663 = local write "max_step_change"(w695) -> ()
        n664 = local write "max_amplitude"(w694) -> ()
        n665 = local write "min_amplitude"(w693) -> ()
        n666 = local write "startup_cmd"(w692) -> ()
      }
    }
    n667 = local read "Quit"() -> (w674:bool)
  }
  n668 = while {
    shift-right: [w729] -> _
    shift-left: "Enum - Selector" -> [w730]
    stop <- w731 stop-if-true
    # "Auto Start Logic Loop"
    n669 = case shown="\"Humidity & Temperature On\"" w730 {
      tunnel: [w734 w740 w767 w799 w829 Auto_Start_enum."Exit" ("Enum - Selector") Auto_Start_enum."Init" ("Enum - Selector")] -> w729
      frame "Init", Default {
        n670 = local read "Auto Start Test"() -> (w733:bool)
        n671 = Select(t=Auto_Start_enum."Humidity & Temperature On" ("Enum - Selector"), s=w733, f=Auto_Start_enum."Init") -> (s? t:f=w734:T15)
      }
      frame "Humidity & Temperature On" {
        n672 = stacked-sequence {
          tunnel: [_ _ _ _ _ _ Auto_Start_enum."Reach point" ("Enum - Selector")] -> w737
          frame #0 {
            w742 = T19."Disabled and Grayed Out" ("Disabled")
            w743 = TRUE ("Heater Button")
            n673 = property on="Humidity" class="Bool (strict)"("DisabledEnum"=w742) -> ()  [unwired: 2 in, 2 out]
            n674 = property on="Heater Button" class="Bool (strict)"("DisabledEnum"=w742) -> ()  [unwired: 2 in, 2 out]
            n675 = local write "Heater Button"(w743) -> ()
            n676 = local write "Humidity"(w743) -> ()
            n677 = property on="Heater Button" class="Bool (strict)"("Val(Sgnl)"=TRUE ("Value (Signaling)")) -> ()  [unwired: 2 in, 2 out]
          }
          frame #1 {
            n678 = Wait (ms)(milliseconds to wait=u32 3000) -> ()  [unwired: 1 out]
          }
          frame #2 {
            n679 = local read "Set Temp"() -> (w749:dbl)
            n680 = Number To Fractional String(number=w749, precision (6)=i16 2) -> (F-format string=w746:string)  [unwired: 2 in]
            n681 = Concatenate Strings("ST;" ("Command"), w746) -> (w747:string)
            n682 = local write "Due Write"(w747) -> ()
          }
          frame #3 {
            n683 = Wait (ms)(milliseconds to wait=u32 1500) -> ()  [unwired: 1 out]
          }
          frame #4 {
            (unwired) i16 2 ("precision (6)")
            n684 = local read "Write UNO"() -> (w751:string[])
            n685 = local read "Set Rh"() -> (w754:dbl)
            n686 = Number To Fractional String(number=w754) -> (F-format string=w755:string)  [unwired: 3 in]
            n687 = Concatenate Strings("M;" ("new element/subarray"), w755) -> (w756:string)
            n688 = local write "Due Write"("HE;1" ("Command")) -> ()
            n689 = Insert Into Array(array=w751, new element=w756) -> (w752:string[])  [unwired: 1 in]
            n690 = local write "Write UNO"(w752) -> ()
          }
          frame #5 {
            n691 = Wait (ms)(milliseconds to wait=u32 1500) -> ()  [unwired: 1 out]
          }
          frame #6 {
            w759 = TRUE ("Reach point temp")
            n692 = local write "Reach point Humidity"(w759) -> ()
            n693 = local write "Reach point temp"(w759) -> ()
          }
        }
        n694 = local read "Auto Start Test"() -> (w739:bool)
        n695 = Not(x=w739) -> (.not. x?=w738:bool)
        n696 = Select(t=Auto_Start_enum."close", s=w738, f=w737) -> (s? t:f=w740:T15)
      }
      frame "Reach point" {
        w768 = TRUE ("PAUSE")
        w776 = 1.0 ("y")
        w779 = 1.0 ("y")
        n697 = local read "Set Temp"() -> (w761:dbl)
        n698 = local read "Set Humidity:"() -> (w775:dbl)
        n699 = local read "Humidity ( %RH )"() -> (w780:dbl)
        n700 = Add(x=w761, y=w779) -> (x+y=w778:dbl)
        n701 = Subtract(x=w761, y=w779) -> (x-y=w777:dbl)
        n702 = Add(x=w775, y=w776) -> (x+y=w774:dbl)
        n703 = Subtract(x=w775, y=w776) -> (x-y=w773:dbl)
        n704 = local read "TEMP"() -> (w781:dbl)
        n705 = In Range and Coerce(upper limit=w774, x=w780, lower limit=w773) -> (In Range?=w762:bool)  [unwired: 1 out]
        n706 = In Range and Coerce(upper limit=w778, x=w781, lower limit=w777) -> (In Range?=w763:bool)  [unwired: 1 out]
        n707 = case shown="True" w762 {
          frame False {
          }
          frame True {
            n708 = case shown="True" "Reach point Humidity" {
              selector: "Reach point Humidity" -> [_ w787]
              frame False {
              }
              frame True {
                n709 = local read "EVENT LOG"() -> (w784:string)
                n710 = Not(x=w787) -> (.not. x?=w786:bool)
                n711 = local write "Reach point Humidity"(w786) -> ()
                n712 = call "Event Log.vi"("Content"="Target Humidity reached", "EVENT LOG"=w784) -> ("EVENT LOG"=w785:string)  [unwired: 8 in, 1 out]
                n713 = local write "EVENT LOG"(w785) -> ()
              }
            }
          }
        }
        n714 = case shown="True" w763 {
          frame False {
          }
          frame True {
            n715 = case shown="True" "Reach point temp" {
              selector: "Reach point temp" -> [_ w793]
              frame False {
              }
              frame True {
                n716 = local read "EVENT LOG"() -> (w790:string)
                n717 = Not(x=w793) -> (.not. x?=w792:bool)
                n718 = local write "Reach point temp"(w792) -> ()
                n719 = call "Event Log.vi"("Content"="Target Temperature reached", "EVENT LOG"=w790) -> ("EVENT LOG"=w791:string)  [unwired: 8 in, 1 out]
                n720 = local write "EVENT LOG"(w791) -> ()
              }
            }
          }
        }
        n721 = local read "Auto Start Test"() -> (w766:bool)
        n722 = And(x=w763, y=w762) -> (x .and. y?=w772:bool)
        n723 = Select(t=Auto_Start_enum."Maintain Stage" ("Enum - Selector"), s=w772, f=Auto_Start_enum."Reach point" ("Enum - Selector")) -> (s? t:f=w769:T15)
        n724 = Not(x=w766) -> (.not. x?=w765:bool)
        n725 = Select(t=Auto_Start_enum."close", s=w765, f=w769) -> (s? t:f=w767:T15)
        n726 = call "ELAPSED TIMER VI.vi"("RESET"=w768, "PAUSE"=w768) -> ()  [unwired: 7 in, 3 out]
      }
      frame "Maintain Stage" {
        w808 = 2.0 ("y")
        w807 = 1.0 ("y")
        # "Humidity and  temperatures Set Point  have been reached"
        n727 = local read "Set Temp"() -> (w794:dbl)
        n728 = local read "Set Humidity:"() -> (w811:dbl)
        n729 = local read "Humidity ( %RH )"() -> (w814:dbl)
        n730 = Add(x=w794, y=w807) -> (x+y=w813:dbl)
        n731 = Subtract(x=w794, y=w807) -> (x-y=w812:dbl)
        n732 = local read "TEMP"() -> (w815:dbl)
        n733 = Add(x=w811, y=w808) -> (x+y=w810:dbl)
        n734 = Subtract(x=w811, y=w808) -> (x-y=w809:dbl)
        n735 = In Range and Coerce(upper limit=w813, x=w815, lower limit=w812) -> (In Range?=w806:bool)  [unwired: 1 out]
        n736 = In Range and Coerce(upper limit=w810, x=w814, lower limit=w809) -> (In Range?=w805:bool)  [unwired: 1 out]
        n737 = And(x=w806, y=w805) -> (x .and. y?=w804:bool)
        n738 = Not(x=w804) -> (.not. x?=w803:bool)
        n739 = call "ELAPSED TIMER VI.vi"("TARGET"=60.0, "RESET"=w803, "PAUSE"=FALSE) -> ("ELAPSED INDICATION"=w800:bool)  [unwired: 6 in, 2 out]
        n740 = case shown="True" w800 {
          tunnel: w800 -> [_ w818]
          tunnel: [Auto_Start_enum."Maintain Stage" ("Enum - Selector") w817] -> w798
          frame False {
          }
          frame True {
            n741 = stacked-sequence {
              tunnel: w818 -> [_ _ _ _ _]
              tunnel: [_ _ _ _ Auto_Start_enum."Start Stage" ("Enum - Selector")] -> w817
              frame #0 {
                n742 = local read "EVENT LOG"() -> (w820:string)
                n743 = call "Event Log.vi"("Content"="Humidity and temperature set point has stabilized.", "EVENT LOG"=w820) -> ("EVENT LOG"=w821:string)  [unwired: 8 in, 1 out]
                n744 = local write "EVENT LOG"(w821) -> ()
              }
              frame #1 {
                n745 = Wait (ms)(milliseconds to wait=u32 100) -> ()  [unwired: 1 out]
              }
              frame #2 {
                n746 = local read "EVENT LOG"() -> (w824:string)
                n747 = call "Event Log.vi"("Content"="Auto Test Started", "EVENT LOG"=w824) -> ("EVENT LOG"=w825:string)  [unwired: 8 in, 1 out]
                n748 = local write "EVENT LOG"(w825) -> ()
              }
              frame #3 {
                w826 = TRUE ("RUN")
                n749 = local write "RUN"(w826) -> ()
                n750 = property on="Auto Start Temp" class="Bool (strict)"("Val(Sgnl)"=w826) -> ()  [unwired: 2 in, 2 out]
                "Auto Start Temp" <- w826
              }
              frame #4 {
              }
            }
          }
        }
        n751 = local read "Auto Start Test"() -> (w797:bool)
        n752 = Not(x=w797) -> (.not. x?=w796:bool)
        n753 = Select(t=Auto_Start_enum."close", s=w796, f=w798) -> (s? t:f=w799:T15)
      }
      frame "Start Stage" {
        w828 = TRUE ("PAUSE")
        n754 = local read "Auto Start Test"() -> (w833:bool)
        n755 = Not(x=w833) -> (.not. x?=w832:bool)
        n756 = Select(t=Auto_Start_enum."close" ("Enum - Selector"), s=w832, f=Auto_Start_enum."Start Stage" ("Enum - Selector")) -> (s? t:f=w829:T15)
        n757 = call "ELAPSED TIMER VI.vi"("RESET"=w828, "PAUSE"=w828) -> ()  [unwired: 7 in, 3 out]
      }
      frame "close" {
        w835 = FALSE ("Heater Button")
        n758 = local write "RUN"(w835) -> ()
        n759 = local write "Heater Button"(w835) -> ()
        n760 = local write "Humidity"(w835) -> ()
        n761 = local write "Auto Start Test"(w835) -> ()
        n762 = property on="Heater Button" class="Bool (strict)"("Val(Sgnl)"=FALSE ("Value (Signaling)")) -> ()  [unwired: 2 in, 2 out]
      }
      frame "Exit" {
      }
    }
    n763 = Wait (ms)(milliseconds to wait=u32 100) -> ()  [unwired: 1 out]
    n764 = local read "Quit"() -> (w731:bool)
  }
  n765 = property on="Service Password Log" class="Str"("Visible"=w21) -> ()  [unwired: 2 in, 2 out]
  n766 = property on="Password 3" class="Clust (strict)"("Visible"=w21) -> ()  [unwired: 2 in, 2 out]
  n767 = while {
    stop <- w864 stop-if-true
    w847 = errorcluster {"status"=FALSE, "code"=0, "source"=""} ("error in (no error) 3")
    # "this loop is for manual report generation"
    n768 = local read "Confirm Measrurement"() -> (w846:bool)
    n769 = case shown="True" w846 {
      selector: w846 -> [_ w954]
      tunnel: errorcluster {"status"=FALSE, "code"=0, "source"=""} ("error in (no error) 3") -> [_ w955]
      tunnel: [_ w953] -> _
      frame False {
      }
      frame True {
        n770 = stacked-sequence {
          tunnel: w955 -> [_ w988 _]
          tunnel: w954 -> [_ _ w1095]
          tunnel: [_ w976 _] -> w953
          frame #0 {
            n771 = String To Path(string="C:\\LAB-IQ\\Image Calibrate v01.dcf") -> (path=w958:path)
            n772 = Open/Create/Replace File ("Open File")(file path (use dialog)=w958) -> (refnum out=w959:refnum<file>)  [unwired: 5 in, 2 out]
            n773 = for {
              N: 4 -> [_]
              tunnel: w959 -> [w965]
              i -> [w961]
              n774 = Read from Text File ("Read File")(file (use dialog)=w965) -> (text=w966:string)  [unwired: 3 in, 3 out]
              n775 = String Subset(string=w966, offset (0)=6, length (rest)=10 ("length (rest)")) -> (substring=w962:string)
              n776 = Fract/Exp String To Number(string=w962) -> (number=w960:dbl)  [unwired: 3 in, 1 out]
              n777 = case shown="3" w961 {
                tunnel: w960 -> [w967 w968 _ w969 _]
                frame 0 {
                  n778 = local write "5x Gain"(w967) -> ()
                }
                frame 1 {
                  n779 = local write "10x Gain"(w968) -> ()
                }
                frame 2 {
                }
                frame 3 {
                  n780 = local write "100x gain"(w969) -> ()
                }
                frame 4, Default {
                }
              }
            }
          }
          frame #1 {
            n781 = local read "TEST STANDARD"() -> (w971:T3)
            n782 = case shown="\"ISO 12156\"" w971 {
              tunnel: ["ASTM D6079" "ISO 12156"] -> w970
              frame "ASTM D6079", Default {
              }
              frame "ISO 12156" {
              }
            }
            n783 = call "IMAGE ANALYSIS.vi"("Enum"=POST_ANALYSIS_ENUM."GET MEASUREMENTS", "error in"=w988) -> ("error out"=w995:errorcluster)  [unwired: 8 in, 1 out]
            n784 = local read "Magnification :"() -> (w981:string)
            n785 = call "Stall Data Flow.vim"("value in"=w995, "milliseconds to wait"=u32 1000) -> ("value out"=w994:errorcluster)  [unwired: 1 out]
            n786 = local read "Test File List :"() -> (w992:string)
            n787 = case shown="\"10x\"" w981 {
              tunnel: [w1031 w1032] -> w979
              frame "5x", Default {
                n788 = local read "5x Gain"() -> (w1031:dbl)
              }
              frame "10x" {
                # "5x"
                n789 = local read "10x Gain"() -> (w1032:dbl)
              }
            }
            n790 = call "IMAGE ANALYSIS.vi"("Enum"=POST_ANALYSIS_ENUM."READ", "error in"=w994) -> ("error out"=w991:errorcluster, "data out"=w982:string)  [unwired: 8 in]
            n791 = Match Pattern(string=w982, regular expression="\"type\": ") -> (after substring=w986:string)  [unwired: 1 in, 3 out]
